vi "UI.vi"(0 "reference in":refnum<class "GUI PumpMotorGroup.lvclass">, 5 "error in (no error)":errorcluster) -> (14 "reference out":refnum<class "GUI PumpMotorGroup.lvclass">, 19 "error out":errorcluster)   [LabVIEW 2019, in "GUI PumpMotorGroup.lvclass"]
uses:
  GUI PumpMotorGroup.lvclass
  C:/Users/ANENKOV_V1/Desktop/SRC_H400/src/GUI_class/GUI.lvclass
  TypeDef/GUI Setting PMG.ctl
  FPGA/TypeDef/blue screan PMG.ctl
  TypeDef/GUI Data Motor.ctl
  TypeDef/State Engine.ctl
  GUI_class/GUI.lvclass/GUI.ctl
  SV_Wrap/SharedVariableWrapper.lvclass/SharedVariableWrapper.ctl
  TypeDef/AI_Data_Array.ctl
  TypeDef/AI_Data.ctl
  TypeDef/AI Statistics Data.ctl
  TypeDef/Data Stand.ctl
  TypeDef/Mode.ctl
  TypeDef/ExecuteStepState.ctl
  TypeDef/Direction.ctl
  Modbus_class/STS REG.ctl
  TypeDef/SP_TYPE.ctl
  TypeDef/State 44-1-2.ctl
  TypeDef/State PMG.ctl
  TypeDef/PMG Mode.ctl
  TypeDef/State Engine 2.ctl
  Modbus_class/CMD REG.ctl
  TypeDef/Active Motor.ctl
  TypeDef/Motor N.ctl
  MessageAMC_class/MessageAMC.lvclass
  C:/Users/ANENKOV_V1/Desktop/SRC_H400/src/MessageInterface_class/MessageInterface.lvclass
  d0ca9bf2-7cd9-4c29-a03d-de1c10393a74.vi
  1340c7c3-4811-47c0-90a3-f070e40b3c2b.vi
  ad647cd1-0ca6-4e2a-9b10-24ebdc4912e3.vi
  ed6eeb3c-dd96-4b8c-8ad6-d0ab6dfe673a.vi
  95c2ceec-78ce-4a4a-9763-a0a2aa26ef74.vi
  ed61e240-b4b4-4ddb-8d5a-21954fee916b.vi
  e9af4671-0cab-4cfc-875a-b0d808fa83ec.vi
  170ed158-a2e2-4c95-ad99-64d454a34a57.vi
  GUI_class/Set Win State.vi
  GUI_class/protected/GetSheredData.vi
  d0ca9bf2-7cd9-4c29-a03d-de1c10393a74.vi/7f19bdff-4430-4bc5-9be5-6ecba5895442.vi
  SV_Wrap/Write Var Info.vi
  SV_Wrap/Read Var Info.vi
  1340c7c3-4811-47c0-90a3-f070e40b3c2b.vi/26ff5948-a1ae-41e5-b59a-0c300c40662b.vi
  ad647cd1-0ca6-4e2a-9b10-24ebdc4912e3.vi/006080e8-d6f1-4322-840c-060899d0e470.vi
  ed6eeb3c-dd96-4b8c-8ad6-d0ab6dfe673a.vi/3ff94406-2fcb-4eb9-8a38-75a53f654a27.vi
  95c2ceec-78ce-4a4a-9763-a0a2aa26ef74.vi/532b5b2b-0f94-4582-9561-62e209be14d2.vi
  ed61e240-b4b4-4ddb-8d5a-21954fee916b.vi/70700920-6ef0-47d6-97fb-f9971d6dfe20.vi
  e9af4671-0cab-4cfc-875a-b0d808fa83ec.vi/7614dc84-a43f-4ebd-bdc1-1b744829c978.vi
  SV_Wrap/Read connection str.vi
  <userlib>/_OpenG.lib/time/time.llb/Tick Count (ms)__ogtk.vi
  GUI_class/GUI.lvclass
  MessageInterface_class/MessageInterface.lvclass
  SV_Wrap/SharedVariableWrapper.lvclass
panel:
  out "String 3":string
  out "String 2":string
  in  "stop pumps":bool
  out "dut":bool
  out "cmber":bool
  out "dt [ms]":u32
  in  "fil chamber":bool
  in  "fil dut":bool
  out "m24":T1 caption="НС очистки и охлаждения"
  out "m21":T1 caption="НС подачи масла"
  out "m12":T1 caption="НС перекачки в бак подачи"
  in  "Stop M24":bool
  in  "Stop M21":bool
  in  "Stop M12":bool
  in  "Activate M24":bool
  in  "Activate M21":bool
  in  "Activate M12":bool
  out "blue screan":T3={"AI1"={"Numeric"=42.780748663101605, "Numeric"=31.016042780748666, "Numeric"=60.96256684491979}, "AI_0"=57.25190839694657, "AI_2"=41.711229946524064, "AI3"={"Numeric"=57.25190839694657, "Numeric"=41.711229946524064, "Numeric"=78.6096256684492}, "M24"=FALSE, "M24 pipe 1"=FALSE, "M24 pipe 2"=FALSE, "M24 pipe 3"=FALSE, "W 18.2"=FALSE, "W 18.2 pipe 2"=FALSE, "W 18.2 pipe 1"=FALSE, "W 18.2 tank"=FALSE, "M12"=FALSE, "M12 pipe 3"=FALSE, "M12 pipe 1"=FALSE, "M12 pipe 2"=FALSE, "M21"=FALSE, "M21 pipe 1"=FALSE, "M21 pipe 2"=FALSE, "M21 pipe 24"=FALSE, "M21 pipe 3"=FALSE, "W18.1"=FALSE, "W18.1 pipe 1"=FALSE, "W18.1 pipe 2"=FALSE, "W18.1 tank"=FALSE, "AO"=0.0, "Average Oil Level"=0.0} {"Average Oil Level" format="%#.1f"; "AI3" scale=0.0..100.0; "AI1" scale=0.0..100.0 scale format="%#.1f"; "AI_2" scale=0.0..100.0; "AI_0" scale=0.0..100.0}
  in  "Setting":T4 {"fililing voltage [V]" min=0.0 max=10.0 step=1.0; "fililing level %" min=0.0 max=10.0 step=1.0; "delta level" min=0.0 max=10.0 step=1.0; "Temp Close Water M21" min=0.0 max=200.0 step=1.0; "Temp Open Water M21" min=0.0 max=200.0 step=1.0; "Temp Turn OFF M24" min=0.0 max=200.0 step=1.0; "Temp Turn ON M24" min=0.0 max=200.0 step=1.0}
  out "Erorr":bool caption="Подключение"
  in  "stop":bool
  # "НС Охлаждения и отчистки (М24)"
  # "НС Подачи масла (М21)"
  # "НС Перекачки масла (М12)"
  # "Заправка"
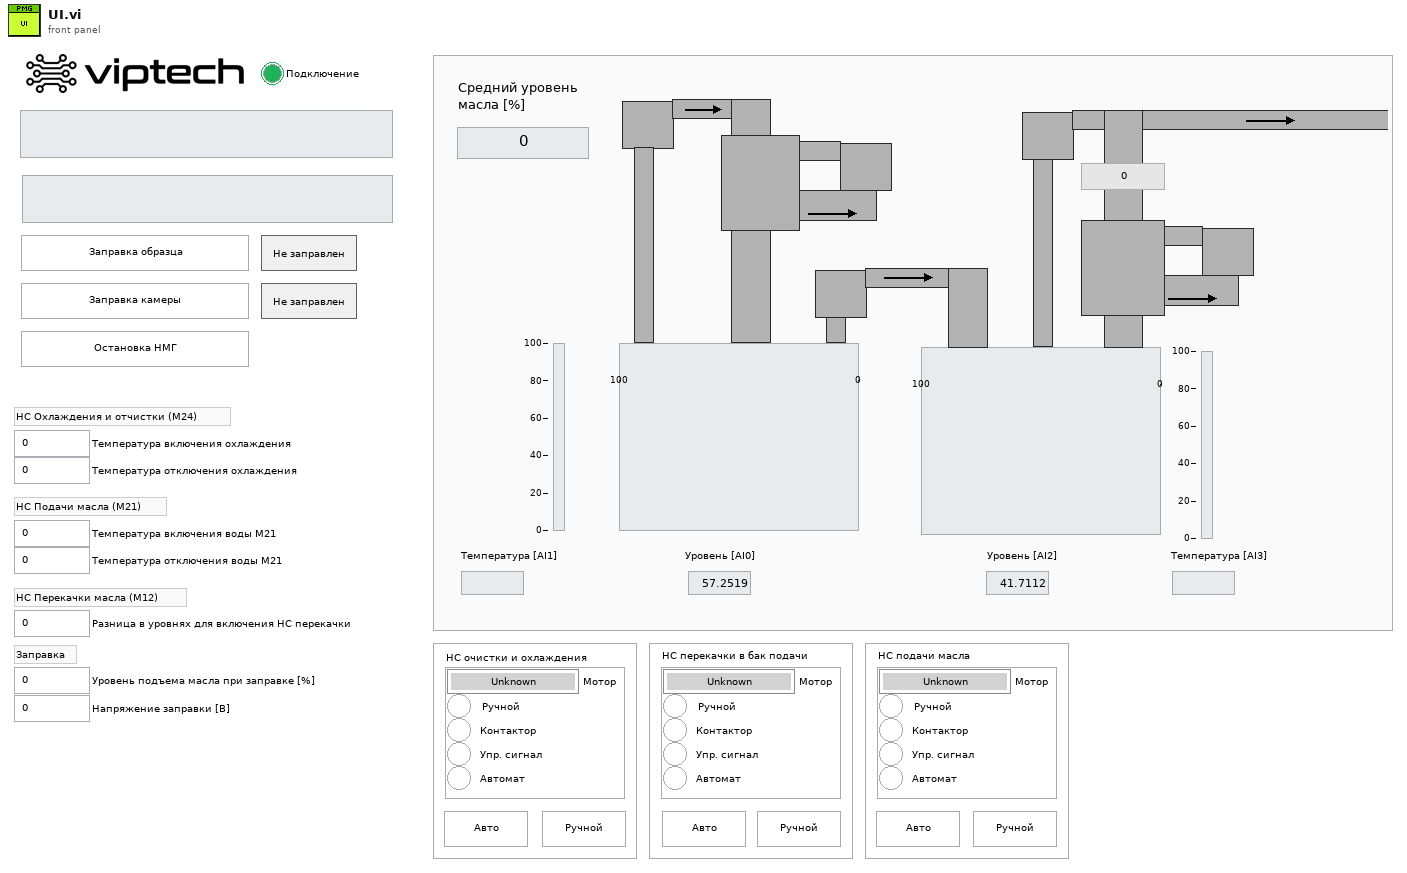
[diagram p1: front panel]
types:
  T1 = typedef "GUI Data Motor.ctl" = cluster{"EngState":T2, "Active":bool, "Contactor":bool, "CMD":bool, "Automat":bool}
  T2 = typedef "State Engine.ctl" = enum16{"Unknown", "Off", "TupningOn", "On", "TurningOff"}
  T3 = typedef "blue screan PMG.ctl" = cluster{"AI1":cluster{"Numeric":dbl, "Numeric":dbl, "Numeric":dbl}, "AI_0":dbl, "AI_2":dbl, "AI3":cluster{"Numeric":dbl, "Numeric":dbl, "Numeric":dbl}, "M24":bool, "M24 pipe 1":bool, "M24 pipe 2":bool, "M24 pipe 3":bool, "W 18.2":bool, "W 18.2 pipe 2":bool, "W 18.2 pipe 1":bool, "W 18.2 tank":bool, "M12":bool, "M12 pipe 3":bool, "M12 pipe 1":bool, "M12 pipe 2":bool, "M21":bool, "M21 pipe 1":bool, "M21 pipe 2":bool, "M21 pipe 24":bool, "M21 pipe 3":bool, "W18.1":bool, "W18.1 pipe 1":bool, "W18.1 pipe 2":bool, "W18.1 tank":bool, "AO":dbl, "Average Oil Level":dbl}
  T4 = typedef "GUI Setting PMG.ctl" = cluster{"Temp Turn ON M24":dbl, "Temp Turn OFF M24":dbl, "Temp Open Water M21":dbl, "Temp Close Water M21":dbl, "delta level":dbl, "fililing level %":dbl, "fililing voltage [V]":dbl}
  T5 = typedef "CMD REG.ctl" = cluster{"EXECUTE_SP":bool, "ALARM_PRESS_DOWN_DUT":bool, "ALARM_PRESS_DOWN_CHAMBER":bool, "ALARM_PRESS_DOWN_DUT_CHAMBER":bool, "FILING_DUT":bool, "FILING_CHAMBER":bool, "BLOCK":bool, "PUMP_STATION_OFF":bool, "Leak start":bool, "Leak stop":bool, "Drain":bool}
  T6 = typedef "Active Motor.ctl" = cluster{"Active":bool, "MotorN":T7}
  T7 = typedef "Motor N.ctl" = enum16{"M12", "M21", "M24"}
  T8 = enum32{"Invalid", "Standard", "Closed", "Hidden", "Minimized", "Maximized"}
  T9 = enum32{"invalid app kind", "Development System", "Run Time System", "Student Edition", "Embedded LabVIEW", "Evaluation", "Custom"}
  T10 = typedef "SharedVariableWrapper.lvclass/Config.ctl" = cluster{"connection str":string, "timeout":dbl, "ip":string}
  T11 = cluster{"Core":cluster{"Current VI Reference":refnum<vi>, "Close Panel on Exit?":bool}, "amc":refnum<class "MessageAMC.lvclass">, "receiver process":string}
  T12 = cluster{"Current VI Reference":refnum<vi>, "Close Panel on Exit?":bool}
  T13 = typedef "AI_Data_Array.ctl" = T14[]
  T14 = typedef "AI_Data.ctl" = cluster{"Stat Data":T15, "OutOfRangeMax":bool, "OutOfRangeMin":bool, "HIHI":bool, "HI":bool, "LO":bool, "LOLO":bool}
  T15 = typedef "AI Statistics Data.ctl" = cluster{"raw mean":dbl, "scl mean":dbl, "raw mean 1Hz":dbl, "scl mean 1Hz":dbl}
  T16 = typedef "Data Stand.ctl" = cluster{"CommCounter":u64, "BeginFilingLevel":dbl, "SP DUT":dbl, "SP CHAMBER":dbl, "Mode":T17, "ExecuteStepState":T18, "Direction":T19, "Direction Filling":T19, "STS":T20, "SP_TYPE_DUT":T21, "SP_TYPE_CHAMBER":T21, "New Step":bool, "BURETE_TIME":u16, "With BURETE":bool, "With Nitro":bool, "State 44-1-2":T22, "Measure leak":bool, "hold":bool}
  T17 = typedef "Mode.ctl" = enum16{"IDLE", "FILLING", "EXECUTE_SP", "DRAIN"}
  T18 = typedef "ExecuteStepState.ctl" = enum16{"Init", "Set: Backpressure ", "Preload: HI", "Set: HI", "Maintenance: HI", "Down: Pressure", "BLOCK"}
  T19 = typedef "Direction.ctl" = enum8{"DUT", "Chamber"}
  T20 = typedef "STS REG.ctl" = cluster{"IDLE":bool, "RYADY":bool, "STEP":bool, "ALARM":bool, "WARNING":bool, "REMOTE":bool, "SP_EXEC_DONE_DUT":bool, "SP_EXEC_DONE_CHAMBER":bool, "FILING_DONE_DUT":bool, "FILING_DONE_CHAMBER":bool, "BURETE_STATE":bool}
  T21 = typedef "SP_TYPE.ctl" = enum16{"ERROR", "ZIRO", "BASE", "SP"}
  T22 = typedef "State 44-1-2.ctl" = enum16{"Init", "Idle", "Wait", "Open 44-1", "Open 44-2", "Close 44-1", "Close 44-2"}
  T23 = typedef "State PMG.ctl" = cluster{"PMG Mode":T24, "M12":T25, "M21":T25, "M24":T25}
  T24 = typedef "PMG Mode.ctl" = enum16{"Idel", "Filling", "Pressure"}
  T25 = typedef "State Engine 2.ctl" = cluster{"EngState":T2, "Active":bool, "Contactor":bool, "CMD":bool, "Automat":bool}
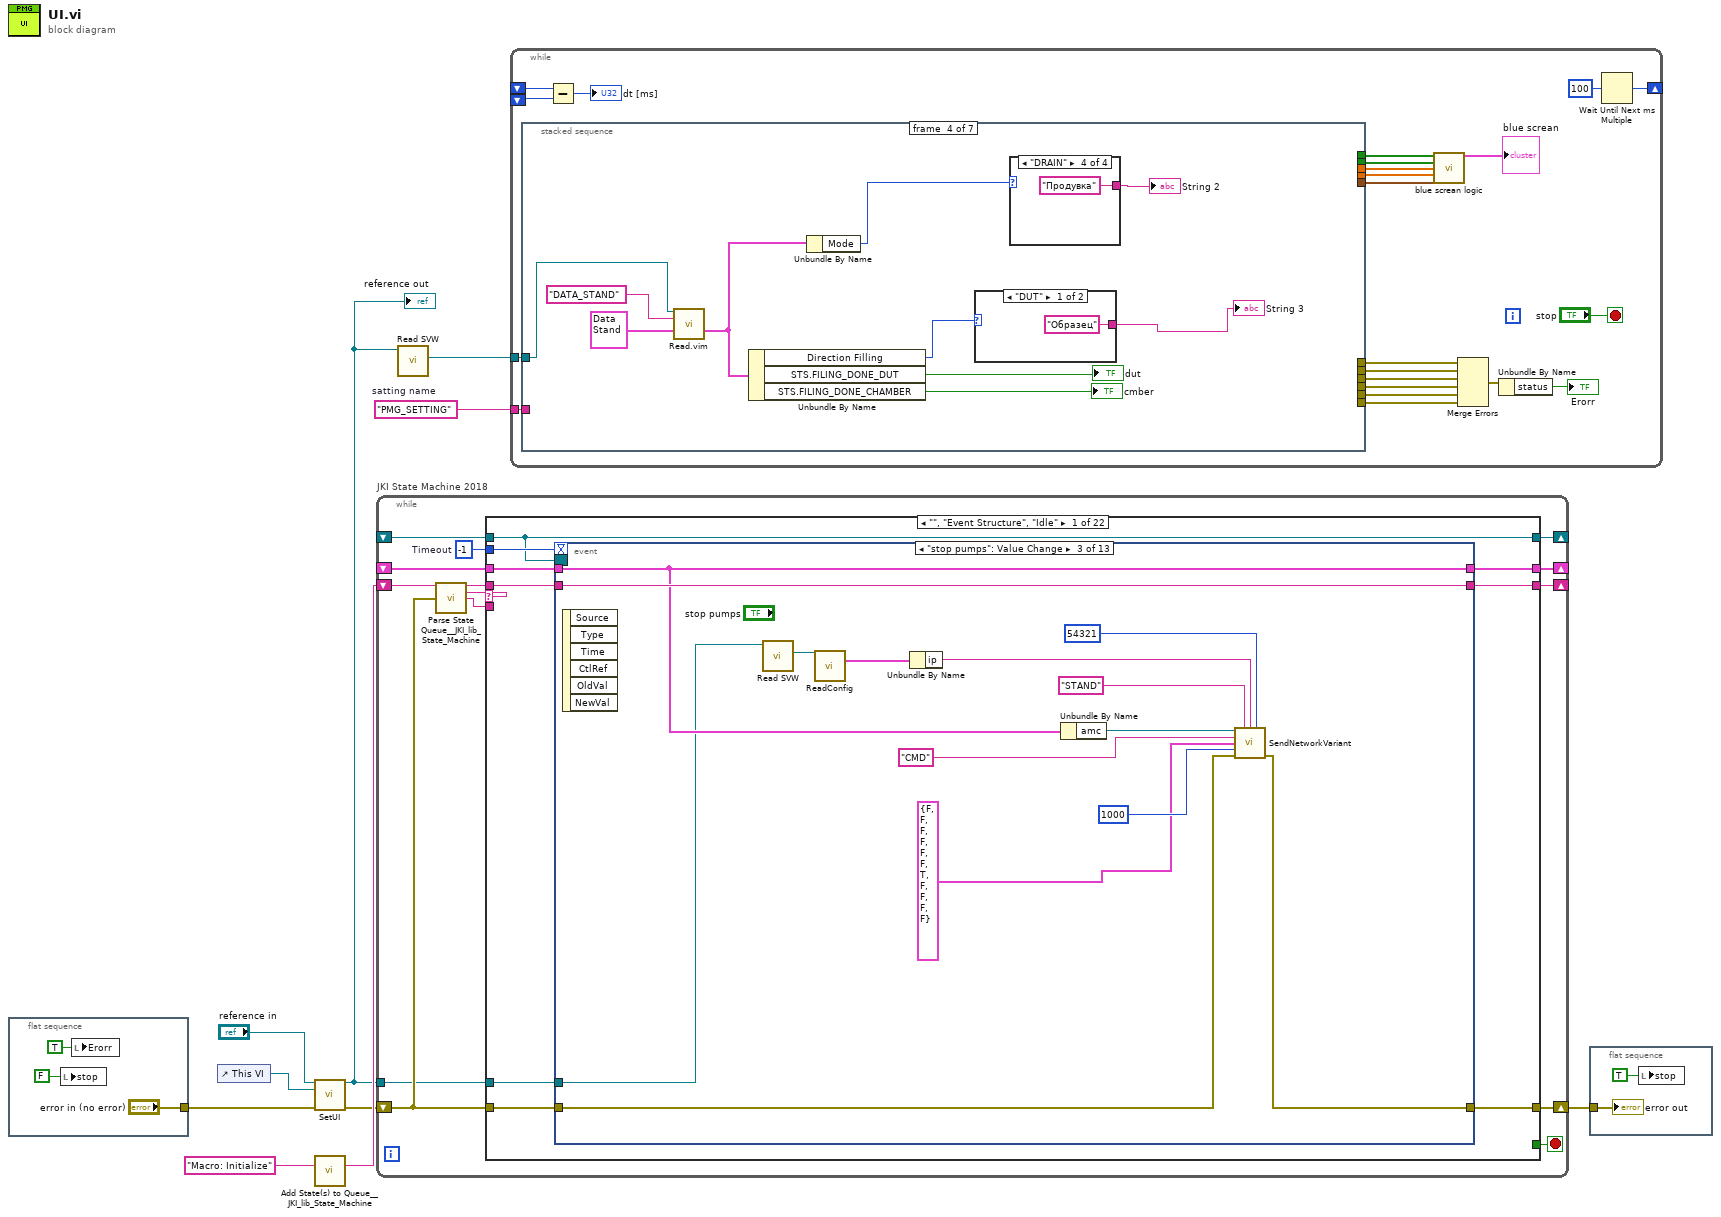
[diagram p0: block diagram]
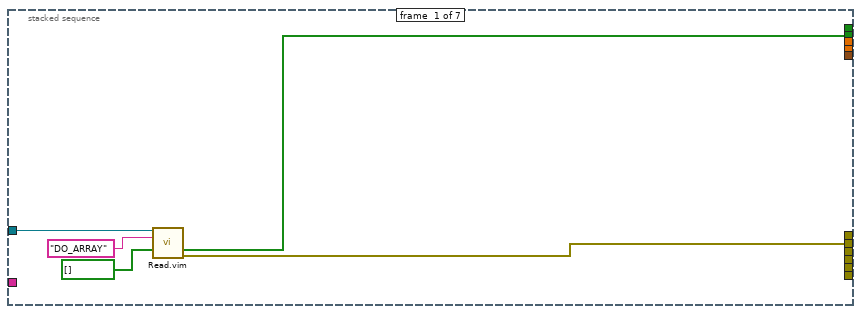
[diagram p2: hidden frame]
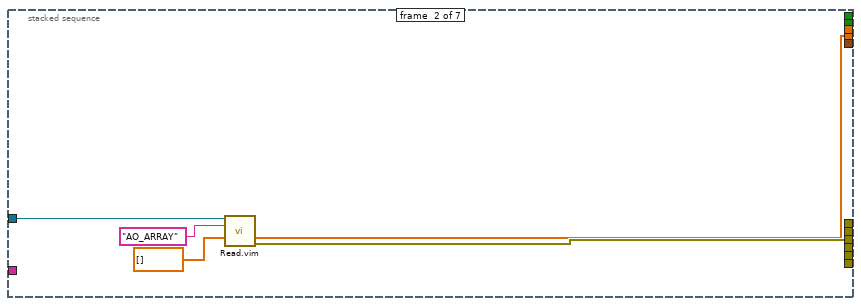
[diagram p3: hidden frame]
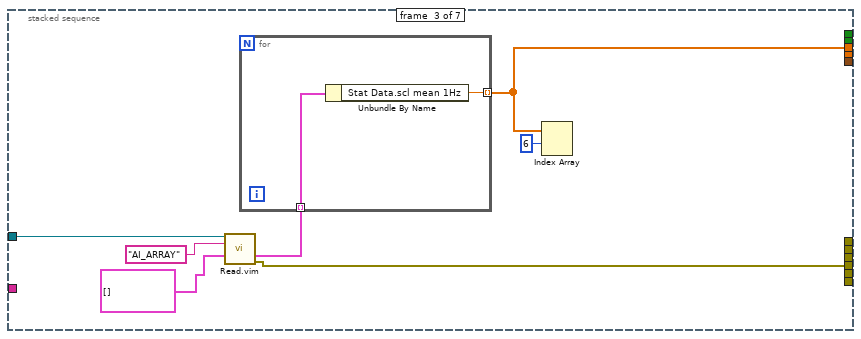
[diagram p4: hidden frame]
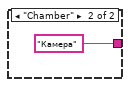
[diagram p5: hidden frame]
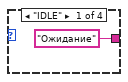
[diagram p6: hidden frame]
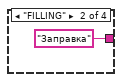
[diagram p7: hidden frame]
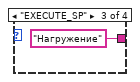
[diagram p8: hidden frame]
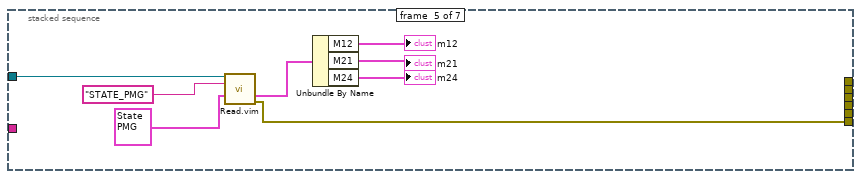
[diagram p9: hidden frame]
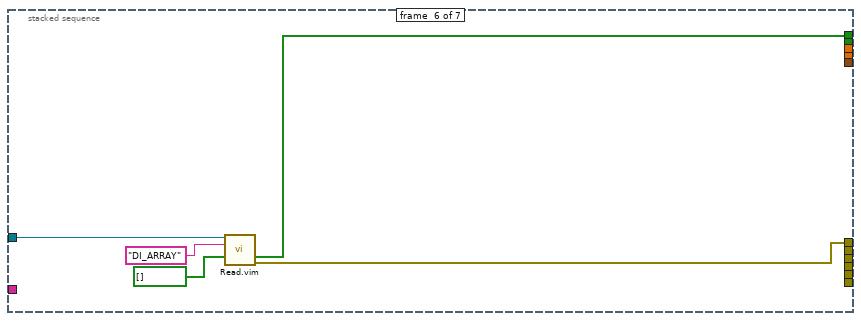
[diagram p10: hidden frame]
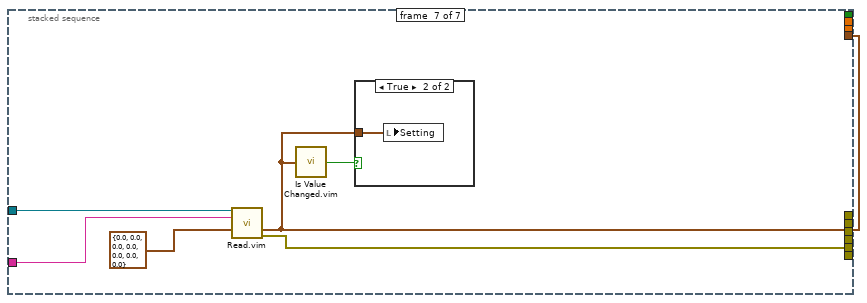
[diagram p11: hidden frame]
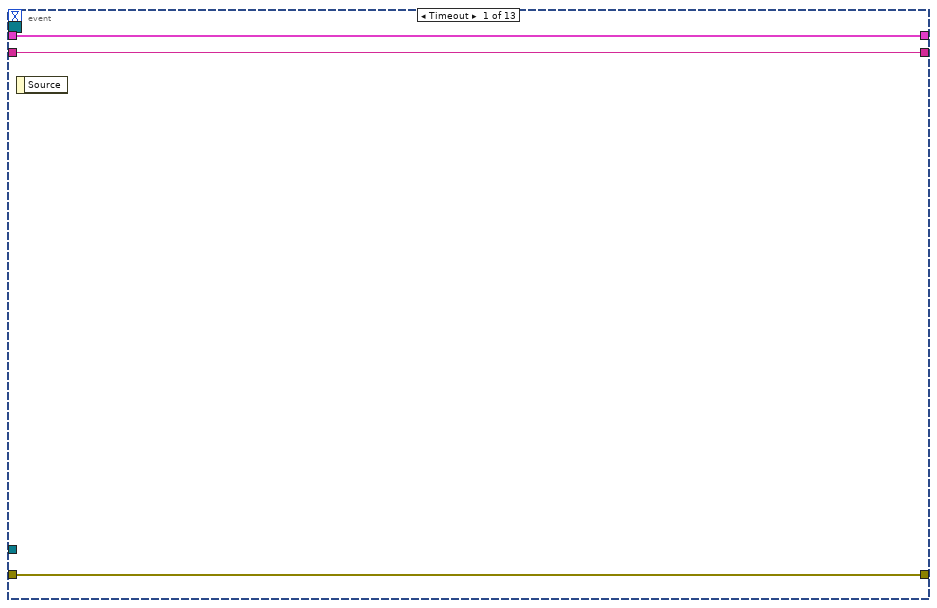
[diagram p13: hidden frame]
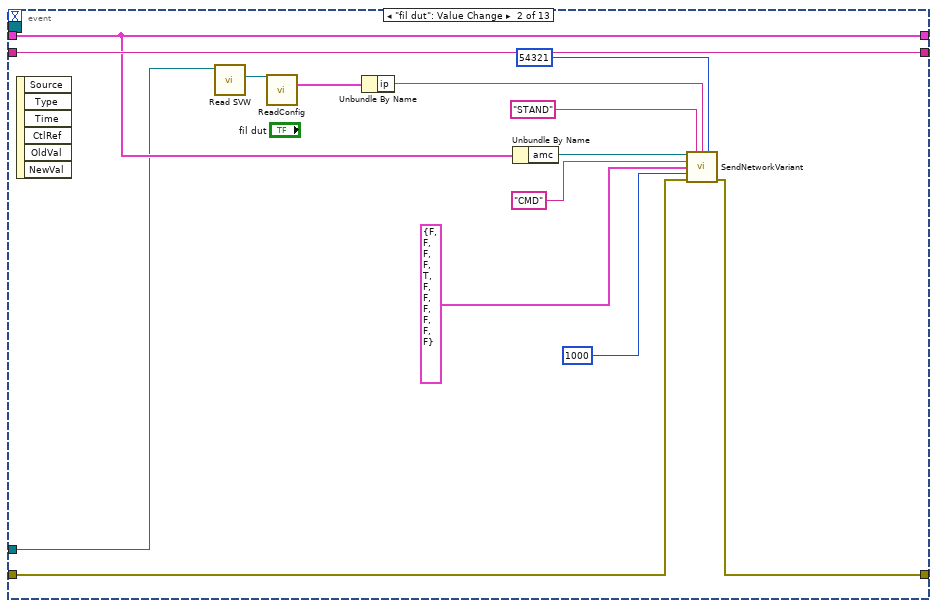
[diagram p14: hidden frame]
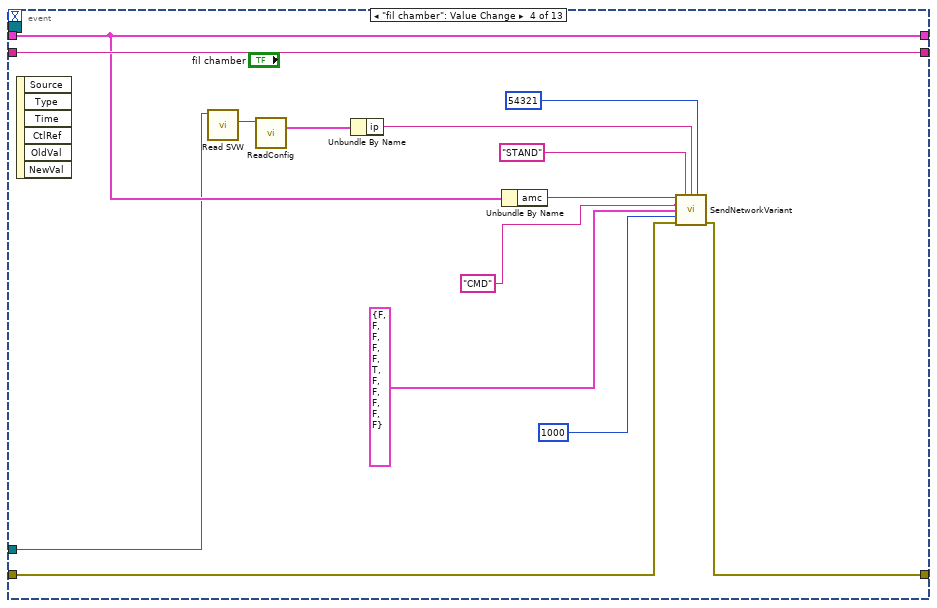
[diagram p15: hidden frame]
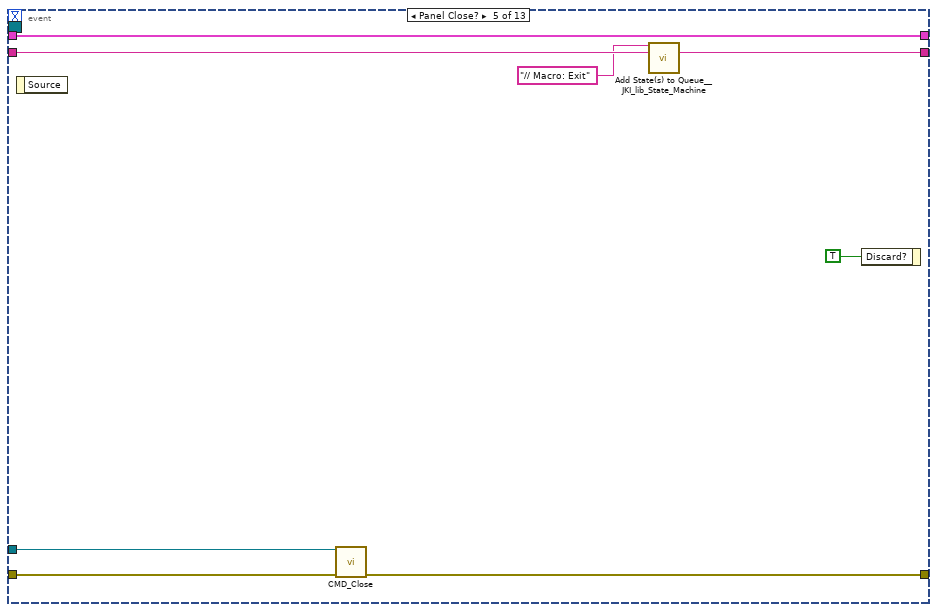
[diagram p16: hidden frame]
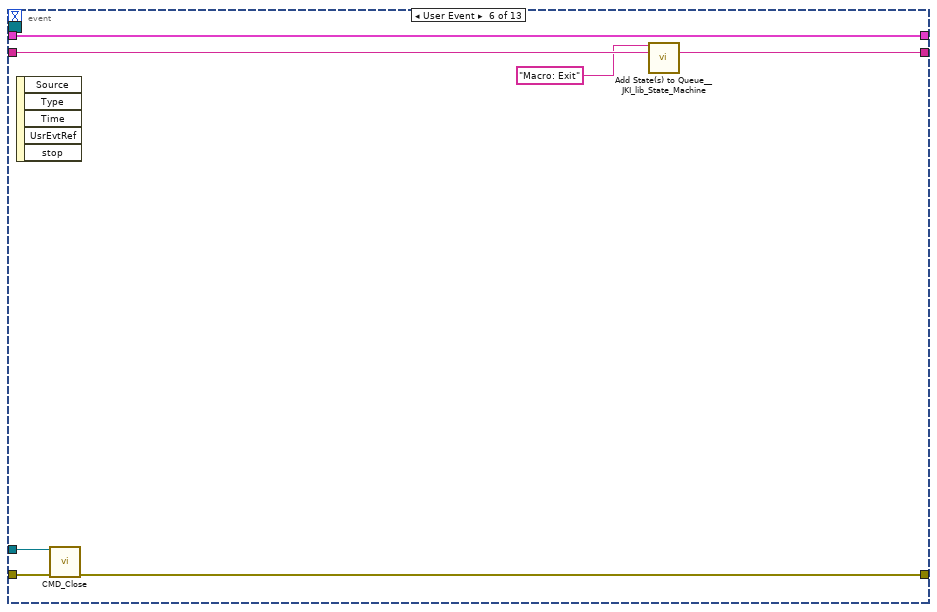
[diagram p17: hidden frame]
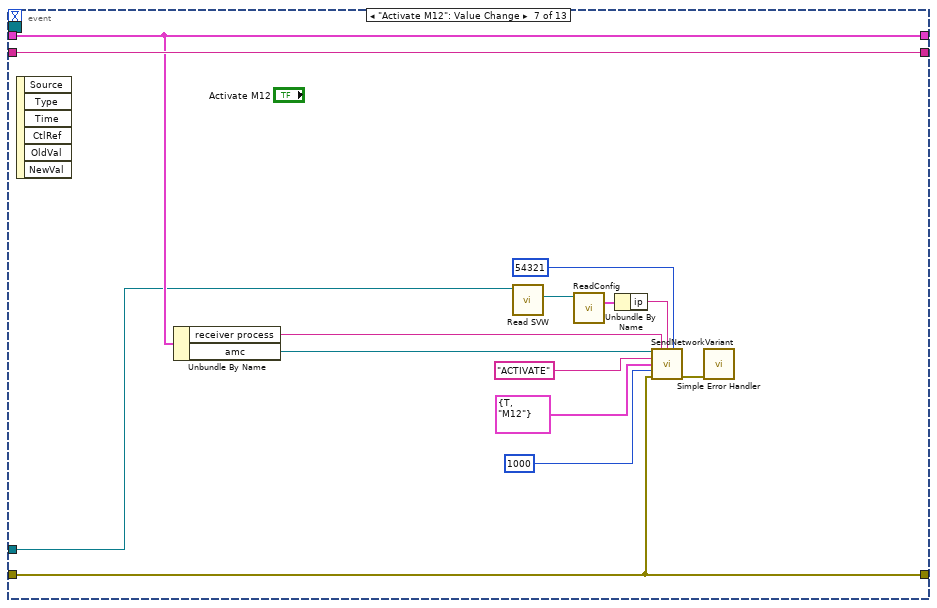
[diagram p18: hidden frame]
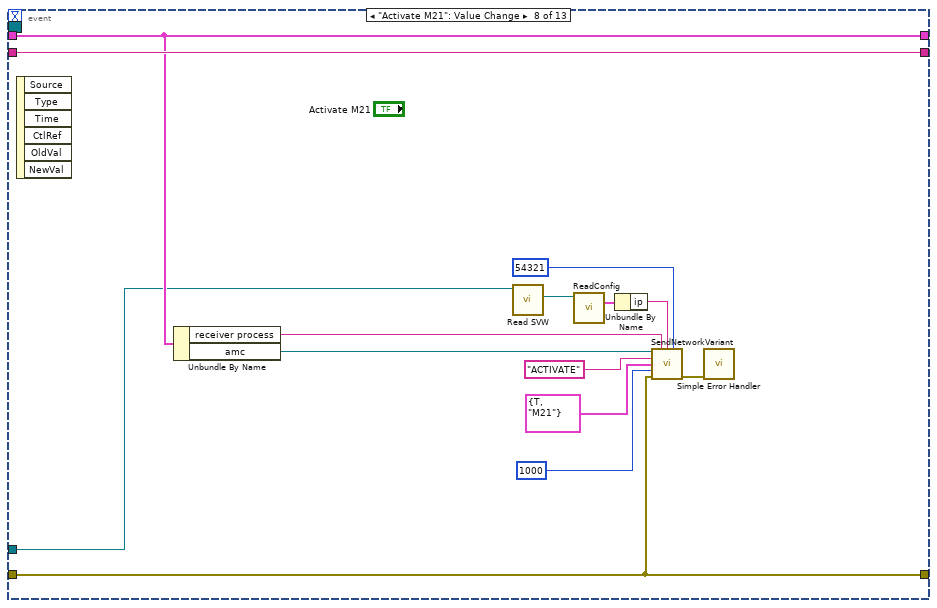
[diagram p19: hidden frame]
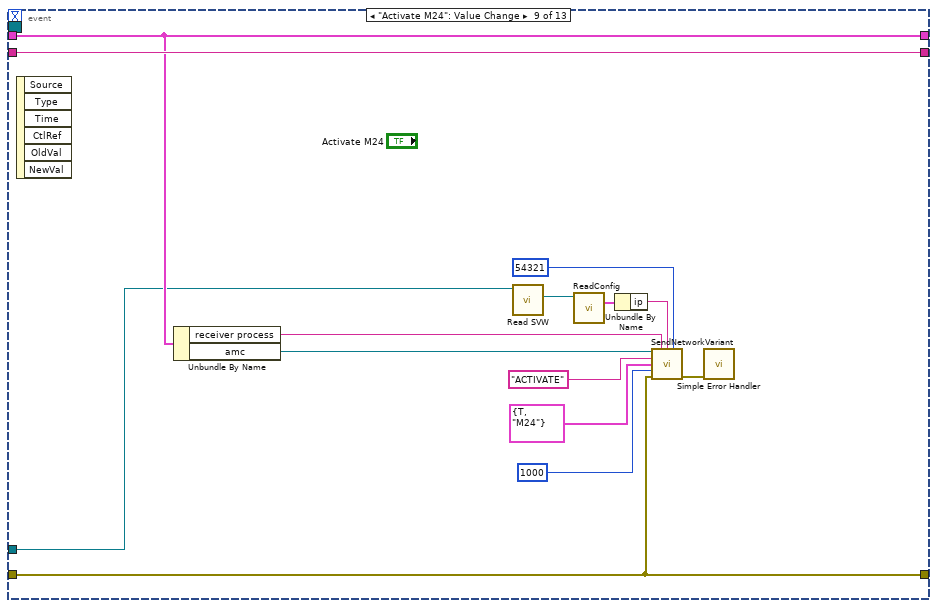
[diagram p20: hidden frame]
diagram:
  w1 = "PMG_SETTING"  # satting name
  n1 = flat-sequence {
    tunnel: ["error in (no error)"] -> w7
    frame #0 {
      n2 = local write "stop"(FALSE ("stop")) -> ()
      n3 = local write "Erorr"(TRUE ("Erorr")) -> ()
    }
  }
  n4 = control-ref of="This VI"() -> (w5:refnum<vi>)
  n5 = call "SetUI.vi"("reference in"="reference in", "UI VI"=w5, "error in (no error)"=w7) -> ("reference out"=w2:refnum<class "GUI PumpMotorGroup.lvclass">, "error out"=w4:errorcluster)  [unwired: 11 in]
  "reference out" <- w2
  n6 = call <vilib>:"Add State(s) to Queue__JKI_lib_State_Machine.vi"("State(s) in (\"\")"="Macro: Initialize") -> ("States Out"=w10:string)  [unwired: 14 in]
  n7 = while "JKI State Machine 2018" {
    shift-right: [w20] -> _
    shift-left: _ -> [w19]
    shift-right: [w23] -> w8
    shift-left: w4 -> [w17]
    shift-right: [w22] -> _
    shift-left: w10 -> [w24]
    tunnel: w2 -> [w16]
    shift-right: [w15] -> _
    shift-left: _ -> [w14]
    stop <- w21 stop-if-true
    w18 = -1  # Timeout
    n8 = call <vilib>:"Parse State Queue__JKI_lib_State_Machine.vi"("State Queue"=w24, "Error In (no error)"=w17) -> ("Remaining States"=w26:string, "Current State"=w27:string, "Arguments"=w25:string)  [unwired: 11 in]
    n9 = case shown="\"\", \"Event Structure\", \"Idle\"" w27 {
      selector: w27 -> [_ _ w195 _ _ _ _ _ _ _ _ _ _ _ _ _ _ _ _ _ _ _]
      tunnel: w26 -> [w36 w193 w199 w219 w226 w234 w239 w249 w255 w260 w268 w274 w279 w283 w290 w302 w372 w378 w384 w396 w400 w407]
      tunnel: w25 -> [_ _ _ _ _ _ _ _ _ _ _ _ _ _ w285 w296 _ _ _ _ _ _]
      tunnel: w19 -> [w34 w190 w197 w212 w223 w229 w236 _ w251 w257 w267 w272 w276 w282 w288 w298 w369 w375 w381 w393 w398 w402]
      tunnel: [w33 w191 w201 w216 errorcluster {"status"=FALSE, "code"=0, "source"=""} ("error out") w232 w237 w242 w252 w258 w265 w269 w277 w281 w286 w299 w370 w376 w382 w394 w399 w404] -> w23
      tunnel: w17 -> [w32 w191 w200 w216 w222 w232 w237 w243 w253 w258 w264 w270 w277 w281 w287 w300 w370 w376 w382 w394 w399 w405]
      tunnel: [w35 w192 w198 w218 w225 w233 w238 w249 w255 w259 w268 w273 w278 w283 w289 w301 w371 w377 w383 w395 w400 w407] -> w22
      tunnel: [_ _ _ _ _ TRUE _ _ _ _ _ _ _ _ _ _ _ _ _ _ _ _] -> w21
      tunnel: [w31 w190 w197 w217 w223 w229 w236 w248 w251 w257 w267 w272 w276 w282 w288 w298 w369 w375 w381 w393 w398 w402] -> w20
      tunnel: w18 -> [w30 _ _ _ _ _ _ _ _ _ _ _ _ _ _ _ _ _ _ _ _ _]
      tunnel: w16 -> [w29 _ _ _ _ _ _ _ _ _ w263 _ _ _ _ _ _ _ _ _ _ w403]
      tunnel: [w28 w189 w194 w206 w220 w230 w235 w246 w250 w256 w266 w271 w275 w280 w284 w295 w368 w373 w379 w386 w397 w406] -> w15
      tunnel: w14 -> [w28 w189 w194 w206 w220 w230 w235 w246 w250 w256 _ w271 w275 w280 w284 w295 w368 w373 w379 w386 w397 w406]
      frame "", "Event Structure", "Idle" {
        n10 = event shown="[2] \"stop pumps\": Value Change" {
          selector: w28 -> [_ _ _ _ _ _ _ _ _ _ _ _ _]
          dyn-events: _ -> [_ _ _ _ _ _ _ _ _ _ _ _ _]
          timeout: w30 -> [_ _ _ _ _ _ _ _ _ _ _ _ _]
          tunnel: w36 -> [w39 w53 w67 w81 w89 w96 w110 w124 w138 w152 w166 w180 w185]
          tunnel: [w39 w53 w67 w81 w88 w95 w110 w124 w138 w152 w166 w180 w186] -> w35
          tunnel: w34 -> [w37 w45 w59 w73 w87 w94 w104 w119 w133 w147 w161 w175 w187]
          tunnel: [w38 w43 w57 w71 w82 w90 w100 w115 w129 w143 w157 w171 w188] -> w33
          tunnel: w32 -> [w38 w44 w58 w72 w83 w91 w100 w115 w129 w143 w157 w171 w188]
          tunnel: [w37 w45 w59 w73 w87 w94 w104 w119 w133 w147 w161 w175 w187] -> w31
          tunnel: w29 -> [_ w42 w56 w70 w84 w92 w99 w114 w128 w142 w156 w170 _]
          event Timeout {
            n11 = event-data() -> ()  [unwired: 1 in, 1 out]
          }
          event "fil dut": Value Change {
            n12 = event-data() -> ()  [unwired: 1 in, 6 out]
            n13 = call "Read SVW.vi"("GUI in"=w42) -> ("SharedVariableWrapper.lvclass"=w52:refnum<class "SharedVariableWrapper.lvclass">)  [unwired: 10 in]
            n14 = call "ReadConfig.vi"("SharedVariableWrapper in"=w52) -> ("config"=w51:T10)  [unwired: 12 in, 2 out]
            n15 = Unbundle By Name(w51) -> ("ip"=w50:string)
            n16 = Unbundle By Name(w45) -> ("amc"=w49:refnum<class "MessageAMC.lvclass">)
            n17 = call "SendNetworkVariant.vi"("reference in"=w49, "receiver process"="STAND", "receiver host"=w50, "receiver port (0)"=u16 54321, "name"="CMD", "data"=T5 {"EXECUTE_SP"=FALSE, "ALARM_PRESS_DOWN_DUT"=FALSE, "ALARM_PRESS_DOWN_CHAMBER"=FALSE, "ALARM_PRESS_DOWN_DUT_CHAMBER"=FALSE, "FILING_DUT"=TRUE, "FILING_CHAMBER"=FALSE, "BLOCK"=FALSE, "PUMP_STATION_OFF"=FALSE, "Leak start"=FALSE, "Leak stop"=FALSE, "Drain"=FALSE} ("CMD REG"), "timeout (25000 ms)"=1000, "error in (no error)"=w44) -> ("error out"=w43:errorcluster)  [unwired: 5 in, 2 out]
          }
          event "stop pumps": Value Change {
            n18 = event-data() -> ()  [unwired: 1 in, 6 out]
            n19 = call "Read SVW.vi"("GUI in"=w56) -> ("SharedVariableWrapper.lvclass"=w66:refnum<class "SharedVariableWrapper.lvclass">)  [unwired: 10 in]
            n20 = call "ReadConfig.vi"("SharedVariableWrapper in"=w66) -> ("config"=w65:T10)  [unwired: 12 in, 2 out]
            n21 = Unbundle By Name(w65) -> ("ip"=w64:string)
            n22 = Unbundle By Name(w59) -> ("amc"=w63:refnum<class "MessageAMC.lvclass">)
            n23 = call "SendNetworkVariant.vi"("reference in"=w63, "receiver process"="STAND", "receiver host"=w64, "receiver port (0)"=u16 54321, "name"="CMD", "data"=T5 {"EXECUTE_SP"=FALSE, "ALARM_PRESS_DOWN_DUT"=FALSE, "ALARM_PRESS_DOWN_CHAMBER"=FALSE, "ALARM_PRESS_DOWN_DUT_CHAMBER"=FALSE, "FILING_DUT"=FALSE, "FILING_CHAMBER"=FALSE, "BLOCK"=TRUE, "PUMP_STATION_OFF"=FALSE, "Leak start"=FALSE, "Leak stop"=FALSE, "Drain"=FALSE} ("CMD REG"), "timeout (25000 ms)"=1000, "error in (no error)"=w58) -> ("error out"=w57:errorcluster)  [unwired: 5 in, 2 out]
          }
          event "fil chamber": Value Change {
            n24 = event-data() -> ()  [unwired: 1 in, 6 out]
            n25 = call "Read SVW.vi"("GUI in"=w70) -> ("SharedVariableWrapper.lvclass"=w80:refnum<class "SharedVariableWrapper.lvclass">)  [unwired: 10 in]
            n26 = call "ReadConfig.vi"("SharedVariableWrapper in"=w80) -> ("config"=w79:T10)  [unwired: 12 in, 2 out]
            n27 = Unbundle By Name(w79) -> ("ip"=w78:string)
            n28 = Unbundle By Name(w73) -> ("amc"=w77:refnum<class "MessageAMC.lvclass">)
            n29 = call "SendNetworkVariant.vi"("reference in"=w77, "receiver process"="STAND", "receiver host"=w78, "receiver port (0)"=u16 54321, "name"="CMD", "data"=T5 {"EXECUTE_SP"=FALSE, "ALARM_PRESS_DOWN_DUT"=FALSE, "ALARM_PRESS_DOWN_CHAMBER"=FALSE, "ALARM_PRESS_DOWN_DUT_CHAMBER"=FALSE, "FILING_DUT"=FALSE, "FILING_CHAMBER"=TRUE, "BLOCK"=FALSE, "PUMP_STATION_OFF"=FALSE, "Leak start"=FALSE, "Leak stop"=FALSE, "Drain"=FALSE} ("CMD REG"), "timeout (25000 ms)"=1000, "error in (no error)"=w72) -> ("error out"=w71:errorcluster)  [unwired: 5 in, 2 out]
          }
          event Panel Close? {
            n30 = event-data() -> ()  [unwired: 1 in, 1 out]
            n31 = call "CMD_Close.vi"("reference in"=w84, "error in (no error)"=w83) -> ("error out"=w82:errorcluster)  [unwired: 12 in, 1 out]
            n32 = call <vilib>:"Add State(s) to Queue__JKI_lib_State_Machine.vi"("State(s) in Front (\"\")"="// Macro: Exit", "State(s) in (\"\")"=w89) -> ("States Out"=w88:string)  [unwired: 13 in]
            n33 = event-data("Discard?"=TRUE) -> ()  [unwired: 1 in, 1 out]
          }
          event User Event {
            n34 = event-data() -> ()  [unwired: 1 in, 5 out]
            n35 = call "CMD_Close.vi"("reference in"=w92, "error in (no error)"=w91) -> ("error out"=w90:errorcluster)  [unwired: 12 in, 1 out]
            n36 = call <vilib>:"Add State(s) to Queue__JKI_lib_State_Machine.vi"("State(s) in Front (\"\")"="Macro: Exit", "State(s) in (\"\")"=w96) -> ("States Out"=w95:string)  [unwired: 13 in]
          }
          event "Activate M12": Value Change {
            n37 = event-data() -> ()  [unwired: 1 in, 6 out]
            n38 = Unbundle By Name(w104) -> ("receiver process"=w98:string, "amc"=w103:refnum<class "MessageAMC.lvclass">)
            n39 = call "Read SVW.vi"("GUI in"=w99) -> ("SharedVariableWrapper.lvclass"=w106:refnum<class "SharedVariableWrapper.lvclass">)  [unwired: 10 in]
            n40 = call "ReadConfig.vi"("SharedVariableWrapper in"=w106) -> ("config"=w105:T10)  [unwired: 12 in, 2 out]
            n41 = Unbundle By Name(w105) -> ("ip"=w102:string)
            n42 = call "SendNetworkVariant.vi"("reference in"=w103, "receiver process"=w98, "receiver host"=w102, "receiver port (0)"=u16 54321, "name"="ACTIVATE", "data"=T6 {"Active"=TRUE, "MotorN"=enum."M12"} ("Active Motor"), "timeout (25000 ms)"=1000, "error in (no error)"=w100) -> ("error out"=w101:errorcluster)  [unwired: 5 in, 2 out]
            n43 = call <vilib>:"Simple Error Handler.vi"("error in (no error)"=w101) -> ()  [unwired: 4 in, 5 out]
          }
          event "Activate M21": Value Change {
            n44 = event-data() -> ()  [unwired: 1 in, 6 out]
            n45 = Unbundle By Name(w119) -> ("receiver process"=w113:string, "amc"=w118:refnum<class "MessageAMC.lvclass">)
            n46 = call "Read SVW.vi"("GUI in"=w114) -> ("SharedVariableWrapper.lvclass"=w121:refnum<class "SharedVariableWrapper.lvclass">)  [unwired: 10 in]
            n47 = call "ReadConfig.vi"("SharedVariableWrapper in"=w121) -> ("config"=w120:T10)  [unwired: 12 in, 2 out]
            n48 = Unbundle By Name(w120) -> ("ip"=w117:string)
            n49 = call "SendNetworkVariant.vi"("reference in"=w118, "receiver process"=w113, "receiver host"=w117, "receiver port (0)"=u16 54321, "name"="ACTIVATE", "data"=T6 {"Active"=TRUE, "MotorN"=enum."M21"} ("Active Motor"), "timeout (25000 ms)"=1000, "error in (no error)"=w115) -> ("error out"=w116:errorcluster)  [unwired: 5 in, 2 out]
            n50 = call <vilib>:"Simple Error Handler.vi"("error in (no error)"=w116) -> ()  [unwired: 4 in, 5 out]
          }
          event "Activate M24": Value Change {
            n51 = event-data() -> ()  [unwired: 1 in, 6 out]
            n52 = Unbundle By Name(w133) -> ("receiver process"=w127:string, "amc"=w132:refnum<class "MessageAMC.lvclass">)
            n53 = call "Read SVW.vi"("GUI in"=w128) -> ("SharedVariableWrapper.lvclass"=w135:refnum<class "SharedVariableWrapper.lvclass">)  [unwired: 10 in]
            n54 = call "ReadConfig.vi"("SharedVariableWrapper in"=w135) -> ("config"=w134:T10)  [unwired: 12 in, 2 out]
            n55 = Unbundle By Name(w134) -> ("ip"=w131:string)
            n56 = call "SendNetworkVariant.vi"("reference in"=w132, "receiver process"=w127, "receiver host"=w131, "receiver port (0)"=u16 54321, "name"="ACTIVATE", "data"=T6 {"Active"=TRUE, "MotorN"=enum."M24"} ("Active Motor"), "timeout (25000 ms)"=1000, "error in (no error)"=w129) -> ("error out"=w130:errorcluster)  [unwired: 5 in, 2 out]
            n57 = call <vilib>:"Simple Error Handler.vi"("error in (no error)"=w130) -> ()  [unwired: 4 in, 5 out]
          }
          event "Stop M12": Value Change {
            n58 = event-data() -> ()  [unwired: 1 in, 6 out]
            n59 = Unbundle By Name(w147) -> ("receiver process"=w141:string, "amc"=w146:refnum<class "MessageAMC.lvclass">)
            n60 = call "Read SVW.vi"("GUI in"=w142) -> ("SharedVariableWrapper.lvclass"=w149:refnum<class "SharedVariableWrapper.lvclass">)  [unwired: 10 in]
            n61 = call "ReadConfig.vi"("SharedVariableWrapper in"=w149) -> ("config"=w148:T10)  [unwired: 12 in, 2 out]
            n62 = Unbundle By Name(w148) -> ("ip"=w145:string)
            n63 = call "SendNetworkVariant.vi"("reference in"=w146, "receiver process"=w141, "receiver host"=w145, "receiver port (0)"=u16 54321, "name"="ACTIVATE", "data"=T6 {"Active"=FALSE, "MotorN"=enum."M12"} ("Active Motor"), "timeout (25000 ms)"=1000, "error in (no error)"=w143) -> ("error out"=w144:errorcluster)  [unwired: 5 in, 2 out]
            n64 = call <vilib>:"Simple Error Handler.vi"("error in (no error)"=w144) -> ()  [unwired: 4 in, 5 out]
          }
          event "Stop M21": Value Change {
            n65 = event-data() -> ()  [unwired: 1 in, 6 out]
            n66 = Unbundle By Name(w161) -> ("receiver process"=w155:string, "amc"=w160:refnum<class "MessageAMC.lvclass">)
            n67 = call "Read SVW.vi"("GUI in"=w156) -> ("SharedVariableWrapper.lvclass"=w163:refnum<class "SharedVariableWrapper.lvclass">)  [unwired: 10 in]
            n68 = call "ReadConfig.vi"("SharedVariableWrapper in"=w163) -> ("config"=w162:T10)  [unwired: 12 in, 2 out]
            n69 = Unbundle By Name(w162) -> ("ip"=w159:string)
            n70 = call "SendNetworkVariant.vi"("reference in"=w160, "receiver process"=w155, "receiver host"=w159, "receiver port (0)"=u16 54321, "name"="ACTIVATE", "data"=T6 {"Active"=FALSE, "MotorN"=enum."M21"} ("Active Motor"), "timeout (25000 ms)"=1000, "error in (no error)"=w157) -> ("error out"=w158:errorcluster)  [unwired: 5 in, 2 out]
            n71 = call <vilib>:"Simple Error Handler.vi"("error in (no error)"=w158) -> ()  [unwired: 4 in, 5 out]
          }
          event "Stop M24": Value Change {
            n72 = event-data() -> ()  [unwired: 1 in, 6 out]
            n73 = Unbundle By Name(w175) -> ("receiver process"=w169:string, "amc"=w174:refnum<class "MessageAMC.lvclass">)
            n74 = call "Read SVW.vi"("GUI in"=w170) -> ("SharedVariableWrapper.lvclass"=w177:refnum<class "SharedVariableWrapper.lvclass">)  [unwired: 10 in]
            n75 = call "ReadConfig.vi"("SharedVariableWrapper in"=w177) -> ("config"=w176:T10)  [unwired: 12 in, 2 out]
            n76 = Unbundle By Name(w176) -> ("ip"=w173:string)
            n77 = call "SendNetworkVariant.vi"("reference in"=w174, "receiver process"=w169, "receiver host"=w173, "receiver port (0)"=u16 54321, "name"="ACTIVATE", "data"=T6 {"Active"=FALSE, "MotorN"=enum."M24"} ("Active Motor"), "timeout (25000 ms)"=1000, "error in (no error)"=w171) -> ("error out"=w172:errorcluster)  [unwired: 5 in, 2 out]
            n78 = call <vilib>:"Simple Error Handler.vi"("error in (no error)"=w172) -> ()  [unwired: 4 in, 5 out]
          }
          event Value Change {
            n79 = event-data() -> ("NewVal"=w183:T4, "OldVal"=w181:T4)  [unwired: 1 in]
            n80 = call "Corect settings.vi"("NewVal"=w183, "OldVal"=w181) -> ("Setting PMG"=w182:T4)  [unwired: 13 in]
            n81 = local write "Setting"(w182) -> ()
            n82 = call <vilib>:"Add State(s) to Queue__jki_lib_state_machine.vi"("State(s) in Front (\"\")"="Action: Write Config" ("State(s) in Front (\"\")"), "State(s) in (\"\")"=w185) -> ("States Out"=w186:string)  [unwired: 13 in]
          }
        }
      }
      frame "---------- Core ----------" {
        n83 = call <vilib>:"Add State(s) to Queue__JKI_lib_State_Machine.vi"("State(s) in (\"\")"=w193) -> ("States Out"=w192:string)  [unwired: 14 in]
      }
      frame Default {
        w204 = 42 items=["No error", "Argument error", "Memory is full", "Out of zone", "End of file", "File already open", "Generic file I/O error", "File not found", "File permission error", "Disk is full", "Duplicate path", "Too many files open", "System feature not enabled", "Resource file not found", "Cannot add resource", "Resource not found", "Image not found", "Image memory error", "Pen does not exist", "Config type invalid", "Config token not found", "Config parse error", "Config memory error", "Bad external code format", "Bad external code offset", "External code not present", "Null window", "Destroy window error", "Null menu", "Print aborted", "Bad print record", "Print driver error", "Windows error during printing", "Memory error during printing", "Print dialog error", "Generic print error", "Invalid device refnum", "Device not found", "Device parameter error", "Device unit error", "Cannot open device", "Device call aborted", "Generic error", "Cancelled by user", "Object ID too low", "Object ID too high", "Object not in heap", "Unknown heap", "Unknown object (invalid DefProc)", "Unknown object (DefProc not in table)", "Message out of range", "Invalid (null) method", "Unknown message", "Manager call not supported", "Bad address", "Network operation in progress", "Network operation timed out", "Connection is busy", "Network attribute not supported", "Network error", "Address in use", "System out of memory", "Connection aborted", "Connection refused", "Not connected", "Already connected", "Connection closed", "Initialization error (interapplication manager)", "Bad occurrence", "Wait on unbound occurrence handler", "Occurrence queue overflow", "Datalog type conflict", "Unused", "Unrecognized type (interapplication manager)", "Memory corrupt", "Failed to make temporary DLL", "Old CIN version", "Drag socket not found", "Failed to load drop-object", "Failed to register OLE object", "Failed to release OLE object", "Format specifier type mismatch", "Unknown format specifier", "Too few format specifiers", "Too many format specifiers", "Scan failed", "Newer CIN version", "Error converting to variant", "Runtime menu error", "Password tampered", "Variant attribute not found", "Incompatible variant data type", "Event data is not available", "Event Store is not present", "Occurrence is not found", "Event Queue is not created", "Event info is not available", "Refnum passed is NULL", "Error retrieving Class GUID", "Error retrieving CoClass GUID", "Error retrieving TypeLib GUID.", "Bad built application magic bytes.", "Specific driver is different from the specific driver associated with the Logical Name.", "There is no session opened to the class driver.", "Max Error", "MAX - Error with config objects", "MAX - Error loading configuration", "MAX - Group not supported"]
        # "Current State"
        # "Do not delete, rename, or modify this frame.\n(this is used to capture unhandled states and typos)"
        # "Handle mistyped state name (developer tool)"
        n84 = Format Into String(format string="Software Exception: Unhandled State \"%s\"." ("message"), error in=w200, w195) -> (resulting string=w203:string, error out=w202:errorcluster)  [unwired: 1 in]
        n85 = call <vilib>:"Error Cluster From Error Code.vi"("show call chain? (False)"=TRUE, "error in (no error)"=w202, "error message (\"\")"=w203, "error code (0)"=w204) -> ("error out"=w201:errorcluster)  [unwired: 5 in]
        n86 = call <vilib>:"Add State(s) to Queue__JKI_lib_State_Machine.vi"("State(s) in (\"\")"=w199) -> ("States Out"=w198:string)  [unwired: 14 in]
      }
      frame "Initialize Core Data" {
        # "Do not delete, rename, or modify this frame.\n(this is used to determine panel behavior on exit)"
        # "originally closed?"
        # "exe?"
        # "If panel starts closed or is an EXE, then close it when we exit"
        n87 = property class="VI"() -> ("FP.State"=w209:T8)  [unwired: 2 in, 2 out]
        n88 = property class="App"() -> ("App.Kind"=w215:T9)  [unwired: 2 in, 2 out]
        n89 = control-ref of="Current VI Reference"() -> (w210:refnum<vi>)
        n90 = Equal?(x=w209, y=T8."Closed" ("Front Panel Window:State")) -> (x = y?=w207:bool)
        n91 = Equal?(x=w215, y=T9."Run Time System" ("Application:Kind")) -> (x = y?=w213:bool)
        n92 = Or(x=w207, y=w213) -> (x .or. y?=w211:bool)
        n93 = Bundle By Name(cluster=w212, "Core.Current VI Reference"=w210, "Core.Close Panel on Exit?"=w211) -> (w217:T11)
        n94 = call <vilib>:"Add State(s) to Queue__JKI_lib_State_Machine.vi"("State(s) in (\"\")"=w219) -> ("States Out"=w218:string)  [unwired: 14 in]
      }
      frame "Error Handler" {
        # "Unhandled Error -- Display it"
        # "Clear error"
        n95 = call <vilib>:"General Error Handler.vi"("error in (no error)"=w222) -> ()  [unwired: 10 in, 5 out]
        n96 = call <vilib>:"Add State(s) to Queue__JKI_lib_State_Machine.vi"("State(s) in Front (\"\")"="/* Post Error States", "State(s) in (\"\")"=w226) -> ("States Out"=w225:string)  [unwired: 13 in]
      }
      frame "Exit" {
        n97 = Unbundle By Name(w229) -> ("amc"=w228:refnum<class "MessageAMC.lvclass">)
        n98 = call-dynamic "Destroy.vi"("reference in"=w228) -> ("error out"=w227:errorcluster)  [unwired: 17 in, 1 out]
        n99 = call <vilib>:"Clear Errors.vi"("error in (no error)"=w227) -> ()  [unwired: 5 in, 2 out]
        n100 = call <vilib>:"Add State(s) to Queue__JKI_lib_State_Machine.vi"("State(s) in (\"\")"=w234) -> ("States Out"=w233:string)  [unwired: 14 in]
      }
      frame "---------- Data ----------" {
        # "Do not put any code in this frame.\n(It is a separator no-op. You can make a copy of this frame to create a new Data frame)"
        n101 = call <vilib>:"Add State(s) to Queue__JKI_lib_State_Machine.vi"("State(s) in (\"\")"=w239) -> ("States Out"=w238:string)  [unwired: 14 in]
      }
      frame "Data: Initialize" {
        w240 = "PMG"  # receiver process
        w247 = T12 {"Current VI Reference"=refnum, "Close Panel on Exit?"=FALSE}  # Core
        n102 = call "MessageAMC_Create.vi"("reference in"=refnum<class "MessageAMC.lvclass"> refnum, "error in (no error)"=w243, "message queue name"="GUI_PMG") -> ("amc"=w244:refnum<class "MessageAMC.lvclass">, "error out"=w242:errorcluster)  [unwired: 15 in]
        n103 = Bundle("Core"=w247, "amc"=w244, "receiver process"=w240) -> (w248:T11)  [unwired: 1 in]
      }
      frame "Data: Cleanup" {
        n104 = Unbundle By Name(w251) -> ("Core.Current VI Reference"=w254:refnum<vi>)
        n105 = Close Reference(reference=w254, error in (no error)=w253) -> (error out=w252:errorcluster)
      }
      frame "---------- Events ----------" {
        # "Do not put any code in this frame.\n(It is a separator no-op. You can make a copy of this frame to create a new UI frame)"
        n106 = call <vilib>:"Add State(s) to Queue__JKI_lib_State_Machine.vi"("State(s) in (\"\")"=w260) -> ("States Out"=w259:string)  [unwired: 14 in]
      }
      frame "Events: Register" {
        n107 = call "Read stop event.vi"("GUI in"=w263) -> ("cmd event"=w261:refnum<user-event>, "stop event"=w262:refnum<user-event>)  [unwired: 8 in, 1 out]
        n108 = register-events(error in=w264, w262, w261) -> (reference out=w266:refnum<event-registration>, error out=w265:errorcluster)  [unwired: 1 in]
      }
      frame "Events: Unregister" {
        # "Do not put any code in this frame.\n(It is a separator no-op. You can make a copy of this frame to create a new UI frame)"
        n109 = Unregister For Events(event registration refnum=w271, error in=w270) -> (error out=w269:errorcluster)
        n110 = call <vilib>:"Add State(s) to Queue__JKI_lib_State_Machine.vi"("State(s) in (\"\")"=w274) -> ("States Out"=w273:string)  [unwired: 14 in]
      }
      frame "---------- UI ----------" {
        # "Do not put any code in this frame.\n(It is a separator no-op. You can make a copy of this frame to create a new UI frame)"
        n111 = call <vilib>:"Add State(s) to Queue__JKI_lib_State_Machine.vi"("State(s) in (\"\")"=w279) -> ("States Out"=w278:string)  [unwired: 14 in]
      }
      frame "UI: Initialize" {
      }
      frame "UI: Cursor Set" {
        # "Argument"
        # "Set and Unset Cursor Busy.\n(Usage: \"UI: Cursor Set >> Busy|Idle\")"
        n112 = case shown="\"Idle\", Default" w285 {
          tunnel: w287 -> [w292 w294]
          tunnel: [w291 w293] -> w286
          frame "Idle", Default {
            n113 = call <vilib>:"Unset Busy.vi"("error in (no error)"=w292) -> ("error out"=w291:errorcluster)  [unwired: 10 in]
          }
          frame "Busy" {
            n114 = call <vilib>:"Set Busy.vi"("error in (no error)"=w294) -> ("error out"=w293:errorcluster)  [unwired: 9 in, 1 out]
          }
        }
        n115 = call <vilib>:"Add State(s) to Queue__JKI_lib_State_Machine.vi"("State(s) in (\"\")"=w290) -> ("States Out"=w289:string)  [unwired: 14 in]
      }
      frame "UI: Front Panel State" {
        # "Argument"
        # "Set Front Panel Open or Closed\n(Usage: \"UI: Front Panel State >> Open|Close\")"
        n116 = Unbundle By Name(w298) -> ("Core.Current VI Reference"=w297:refnum<vi>)
        n117 = case shown="\"Minimize\", \"Minimized\"" w296 {
          tunnel: w300 -> [w308 w323 w334 w347 w360]
          tunnel: [w310 w324 w336 w349 w362] -> w299
          tunnel: w297 -> [w309 w321 w335 w348 w361]
          frame "Open", "Standard", Default {
            w303 = T8."Standard" ("State")
            n118 = property class="VI"(reference=w309, error in=w308) -> (reference out=w306:refnum<vi>, error out=w307:errorcluster, "FP.State"=w305:T8)
            n119 = Not Equal?(x=w305, y=w303) -> (x != y?=w304:bool)
            n120 = case shown="True" w304 {
              tunnel: [w314 w316] -> w310
              tunnel: w307 -> [w313 w316]
              tunnel: w306 -> [w312 _]
              tunnel: w303 -> [w311 _]
              frame True {
                n121 = invoke class="VI" method="FP.Open"(reference=w312, error in=w313, "Activate"=TRUE, "State"=w311) -> (error out=w314:errorcluster)  [unwired: 1 in, 4 out]
              }
              frame False {
              }
            }
          }
          frame "Close", "Closed" {
            n122 = property class="VI"(reference=w321, error in=w323) -> (reference out=w320:refnum<vi>, error out=w322:errorcluster, "FP.State"=w318:T8)
            n123 = Not Equal?(x=w318, y=T8."Closed" ("Front Panel Window:State")) -> (x != y?=w317:bool)
            n124 = case shown="True" w317 {
              tunnel: [w325 w328] -> w324
              tunnel: w322 -> [w325 w327]
              tunnel: w320 -> [_ w326]
              frame False {
              }
              frame True {
                n125 = invoke class="VI" method="FP.Close"(reference=w326, error in=w327) -> (error out=w328:errorcluster)  [unwired: 1 in, 2 out]
              }
            }
          }
          frame "Hidden", "Hide" {
            w329 = T8."Hidden" ("State")
            n126 = property class="VI"(reference=w335, error in=w334) -> (reference out=w332:refnum<vi>, error out=w333:errorcluster, "FP.State"=w331:T8)
            n127 = Not Equal?(x=w331, y=w329) -> (x != y?=w330:bool)
            n128 = case shown="True" w330 {
              tunnel: [w340 w341] -> w336
              tunnel: w333 -> [w339 w341]
              tunnel: w332 -> [w338 _]
              tunnel: w329 -> [w337 _]
              frame True {
                n129 = invoke class="VI" method="FP.Open"(reference=w338, error in=w339, "State"=w337) -> (error out=w340:errorcluster)  [unwired: 2 in, 4 out]
              }
              frame False {
              }
            }
          }
          frame "Minimize", "Minimized" {
            w342 = T8."Minimized" ("State")
            n130 = property class="VI"(reference=w348, error in=w347) -> (reference out=w345:refnum<vi>, error out=w346:errorcluster, "FP.State"=w344:T8)
            n131 = Not Equal?(x=w344, y=w342) -> (x != y?=w343:bool)
            n132 = case shown="True" w343 {
              tunnel: [w353 w354] -> w349
              tunnel: w346 -> [w352 w354]
              tunnel: w345 -> [w351 _]
              tunnel: w342 -> [w350 _]
              frame True {
                n133 = invoke class="VI" method="FP.Open"(reference=w351, error in=w352, "State"=w350) -> (error out=w353:errorcluster)  [unwired: 2 in, 4 out]
              }
              frame False {
              }
            }
          }
          frame "Maximize", "Maximized" {
            w355 = T8."Maximized" ("State")
            n134 = property class="VI"(reference=w361, error in=w360) -> (reference out=w358:refnum<vi>, error out=w359:errorcluster, "FP.State"=w357:T8)
            n135 = Not Equal?(x=w357, y=w355) -> (x != y?=w356:bool)
            n136 = case shown="True" w356 {
              tunnel: [w366 w367] -> w362
              tunnel: w359 -> [w365 w367]
              tunnel: w358 -> [w364 _]
              tunnel: w355 -> [w363 _]
              frame True {
                n137 = invoke class="VI" method="FP.Open"(reference=w364, error in=w365, "State"=w363) -> (error out=w366:errorcluster)  [unwired: 2 in, 4 out]
              }
              frame False {
              }
            }
          }
        }
        n138 = call <vilib>:"Add State(s) to Queue__JKI_lib_State_Machine.vi"("State(s) in (\"\")"=w302) -> ("States Out"=w301:string)  [unwired: 14 in]
      }
      frame "---------- Macro ----------" {
        # "Do not put any code in this frame.\n(It is a separator no-op. You can make a copy of this frame to create a new Macro frame)"
        n139 = call <vilib>:"Add State(s) to Queue__JKI_lib_State_Machine.vi"("State(s) in (\"\")"=w372) -> ("States Out"=w371:string)  [unwired: 14 in]
      }
      frame "Macro: Initialize" {
        n140 = call <vilib>:"Add State(s) to Queue__JKI_lib_State_Machine.vi"("State(s) in Front (\"\")"="Data: Initialize\nInitialize Core Data\nEvents: Register\nUI: Initialize\n// UI: Front Panel State >> Open\n\n", "State(s) in (\"\")"=w378) -> ("States Out"=w377:string)  [unwired: 13 in]
      }
      frame "Macro: Update" {
        n141 = call <vilib>:"Add State(s) to Queue__JKI_lib_State_Machine.vi"("State(s) in Front (\"\")"="Action: Write Config", "State(s) in (\"\")"=w384) -> ("States Out"=w383:string)  [unwired: 13 in]
      }
      frame "Macro: Exit" {
        # "Exit Macro\n(This is called once, when the VI exits)"
        n142 = Unbundle By Name(w393) -> ("Core.Close Panel on Exit?"=w392:bool)
        n143 = Select(t="UI: Front Panel State >> Close", s=w392, f="") -> (s? t:f=w389:string)
        n144 = call <vilib>:"Add State(s) to Queue__JKI_lib_State_Machine.vi"("State(s) in Front (\"\")"="Action: Write Config", "State(s) in (\"\")"=w389, "State(s) at Back (\"\")"="Data: Cleanup\nEvents: Unregister\nExit") -> ("States Out"=w387:string)  [unwired: 12 in]
        n145 = call <vilib>:"Add State(s) to Queue__JKI_lib_State_Machine.vi"("State(s) in Front (\"\")"=w387, "State(s) in (\"\")"=w396) -> ("States Out"=w395:string)  [unwired: 13 in]
      }
      frame "---------- Action ----------" {
      }
      frame "Action: Write Config" {
        n146 = local read "Erorr"() -> (w401:bool)
        n147 = case shown="False" w401 {
          tunnel: w405 -> [w412 w421]
          tunnel: [w414 w421] -> w404
          tunnel: w403 -> [w411 _]
          tunnel: w402 -> [w410 _]
          frame False {
            n148 = Unbundle By Name(w410) -> ("receiver process"=w409:string, "amc"=w417:refnum<class "MessageAMC.lvclass">)
            n149 = call "Read SVW.vi"("GUI in"=w411) -> ("SharedVariableWrapper.lvclass"=w420:refnum<class "SharedVariableWrapper.lvclass">)  [unwired: 10 in]
            n150 = call "ReadConfig.vi"("SharedVariableWrapper in"=w420) -> ("config"=w419:T10)  [unwired: 12 in, 2 out]
            n151 = Unbundle By Name(w419) -> ("ip"=w418:string)
            n152 = call "SendNetworkVariant.vi"("reference in"=w417, "receiver process"=w409, "receiver host"=w418, "receiver port (0)"=u16 54321, "name"="SET_SETTINGS", "data"="Setting", "timeout (25000 ms)"=1000, "error in (no error)"=w412) -> ("error out"=w414:errorcluster)  [unwired: 5 in, 2 out]
          }
          frame True {
          }
        }
      }
    }
  }
  n153 = call "Read SVW.vi"("GUI in"=w2) -> ("SharedVariableWrapper.lvclass"=w3:refnum<class "SharedVariableWrapper.lvclass">)  [unwired: 10 in]
  n154 = while {
    tunnel: w3 -> [w441]
    tunnel: w1 -> [w426]
    shift-right: [w425] -> _
    shift-left: _ -> [w424]
    shift-left: _ -> [w423]
    stop <- "stop" stop-if-true
    n155 = stacked-sequence {
      tunnel: w441 -> [w448 w453 w460 w470 w486 w491 w496]
      tunnel: [w445 _ _ _ _ _ _] -> w440
      tunnel: [_ _ _ _ _ w488 _] -> w437
      tunnel: [_ _ _ _ _ w487 _] -> w435
      tunnel: [w444 _ _ _ _ _ _] -> w434
      tunnel: [_ w450 _ _ _ _ _] -> w433
      tunnel: [_ w449 _ _ _ _ _] -> w432
      tunnel: [_ _ w458 _ _ _ _] -> w431
      tunnel: [_ _ w455 _ _ _ _] -> w430
      tunnel: [_ _ _ _ _ _ w494] -> w429
      tunnel: [_ _ _ _ _ _ w495] -> w428
      tunnel: [_ _ _ _ w479 _ _] -> w427
      tunnel: w426 -> [_ _ _ _ _ _ w492]
      frame #0 {
        n156 = call "Read.vim"("SharedVariableWrapper in"=w448, "name"="DO_ARRAY", "DataType"=bool[] []) -> ("data out"=w444:bool[], "error out"=w445:errorcluster)  [unwired: 6 in, 5 out]
      }
      frame #1 {
        n157 = call "Read.vim"("SharedVariableWrapper in"=w453, "name"="AO_ARRAY", "DataType"=dbl[] []) -> ("data out"=w449:dbl[], "error out"=w450:errorcluster)  [unwired: 6 in, 5 out]
      }
      frame #2 {
        n158 = call "Read.vim"("SharedVariableWrapper in"=w460, "name"="AI_ARRAY", "DataType"=T13 [] ("AI_Data_Array")) -> ("data out"=w456:T13, "error out"=w458:errorcluster)  [unwired: 6 in, 5 out]
        n159 = for {
          tunnel: w456 -> [w462] mode=indexing
          tunnel: [w461] -> w455 mode=indexing
          n160 = Unbundle By Name(w462) -> ("Stat Data.scl mean 1Hz"=w461:dbl)
        }
        n161 = Index Array(array=w455, index #1=6 ("index")) -> ()  [unwired: 1 in, 2 out]
      }
      frame #3 {
        n162 = call "Read.vim"("SharedVariableWrapper in"=w470, "name"="DATA_STAND", "DataType"=T16 {"CommCounter"=0, "BeginFilingLevel"=0.0, "SP DUT"=0.0, "SP CHAMBER"=0.0, "Mode"=enum."IDLE", "ExecuteStepState"=enum."Init", "Direction"=enum."DUT", "Direction Filling"=enum."DUT", "STS"={"IDLE"=FALSE, "RYADY"=FALSE, "STEP"=FALSE, "ALARM"=FALSE, "WARNING"=FALSE, "REMOTE"=FALSE, "SP_EXEC_DONE_DUT"=FALSE, "SP_EXEC_DONE_CHAMBER"=FALSE, "FILING_DONE_DUT"=FALSE, "FILING_DONE_CHAMBER"=FALSE, "BURETE_STATE"=FALSE}, "SP_TYPE_DUT"=enum."ZIRO", "SP_TYPE_CHAMBER"=enum."ZIRO", "New Step"=FALSE, "BURETE_TIME"=0, "With BURETE"=FALSE, "With Nitro"=FALSE, "State 44-1-2"=enum."Init", "Measure leak"=FALSE, "hold"=FALSE} ("Data Stand")) -> ("data out"=w467:T16)  [unwired: 6 in, 6 out]
        n163 = Unbundle By Name(w467) -> ("Direction Filling"=w464:T19, "STS.FILING_DONE_DUT"=→"dut":bool, "STS.FILING_DONE_CHAMBER"=→"cmber":bool)
        n164 = Unbundle By Name(w467) -> ("Mode"=w466:T17)
        n165 = case shown="\"DUT\"" w464 {
          tunnel: ["Образец" ("format string") "Камера" ("format string")] -> w463
          frame "DUT" {
          }
          frame "Chamber" {
          }
        }
        "String 3" <- w463
        n166 = case shown="\"DRAIN\"" w466 {
          tunnel: ["Ожидание" ("String") "Заправка" ("String") "Нагружение" ("String") "Продувка" ("String")] -> w465
          frame "IDLE" {
          }
          frame "FILLING" {
          }
          frame "EXECUTE_SP" {
          }
          frame "DRAIN" {
          }
        }
        "String 2" <- w465
      }
      frame #4 {
        n167 = call "Read.vim"("SharedVariableWrapper in"=w486, "name"="STATE_PMG", "DataType"=T23 {"PMG Mode"=enum."Idel", "M12"={"EngState"=enum."Unknown", "Active"=FALSE, "Contactor"=FALSE, "CMD"=FALSE, "Automat"=FALSE}, "M21"={"EngState"=enum."Unknown", "Active"=FALSE, "Contactor"=FALSE, "CMD"=FALSE, "Automat"=FALSE}, "M24"={"EngState"=enum."Unknown", "Active"=FALSE, "Contactor"=FALSE, "CMD"=FALSE, "Automat"=FALSE}} ("PMG")) -> ("data out"=w483:T23, "error out"=w479:errorcluster)  [unwired: 6 in, 5 out]
        n168 = Unbundle By Name(w483) -> ("M12"=→"m12":T25, "M21"=→"m21":T25, "M24"=→"m24":T25)
      }
      frame #5 {
        n169 = call "Read.vim"("SharedVariableWrapper in"=w491, "name"="DI_ARRAY", "DataType"=bool[] []) -> ("data out"=w487:bool[], "error out"=w488:errorcluster)  [unwired: 6 in, 5 out]
      }
      frame #6 {
        n170 = call "Read.vim"("SharedVariableWrapper in"=w496, "name"=w492, "DataType"=T4 {"Temp Turn ON M24"=0.0, "Temp Turn OFF M24"=0.0, "Temp Open Water M21"=0.0, "Temp Close Water M21"=0.0, "delta level"=0.0, "fililing level %"=0.0, "fililing voltage [V]"=0.0} ("Setting")) -> ("data out"=w494:T4, "error out"=w495:errorcluster)  [unwired: 6 in, 5 out]
        n171 = call "Is Value Changed.vim"("value"=w494) -> ("changed or first call?"=w493:bool)
        n172 = case shown="True" w493 {
          tunnel: w494 -> [_ w498]
          frame False {
          }
          frame True {
            n173 = local write "Setting"(w498) -> ()
          }
        }
      }
    }
    n174 = Subtract(x=w424, y=w423) -> (x-y=→"dt [ms]":u32)
    n175 = call "blue screan logic.vi"("DI"=w435, "DO"=w434, "AI"=w430, "AO"=w432, "Setting"=w429) -> ("blue screan PMG"=→"blue screan":T3)  [unwired: 10 in]
    n176 = Merge Errors(w437, w440, w433, w431, w428, w427) -> (w439:errorcluster)
    n177 = Unbundle By Name(w439) -> ("status"=→"Erorr":bool)
    n178 = Wait Until Next ms Multiple(millisecond multiple=u32 100) -> (millisecond timer value=w425:u32)
  }
  n179 = flat-sequence {
    tunnel: w8 -> [w500]
    frame #0 {
      n180 = local write "stop"(TRUE ("stop")) -> ()
      "error out" <- w500
    }
  }
